vi "write.vi"(8 "error in (no error)":errorcluster, 10 "writeString":string, 11 "SerialReal in":refnum<class "SerialReal.lvclass">) -> (0 "error out":errorcluster, 3 "SerialReal out":refnum<class "SerialReal.lvclass">)   [LabVIEW 2013, in "SerialProtocols.lvlib" / "SerialReal.lvclass"]
uses:
  <userlib>/Common/SerialProtocols/SerialCommunicator/SerialReal/SerialReal.lvclass
  <userlib>/Common/SerialProtocols/SerialCommunicator/SerialReal/SerialReal.lvclass/SerialReal.ctl
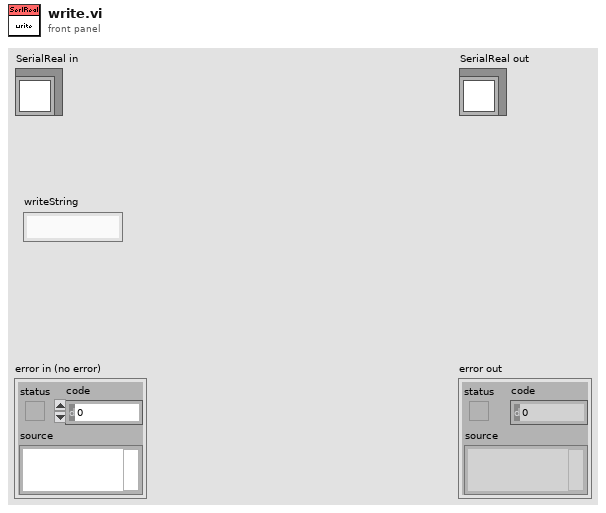
[diagram p1: front panel]
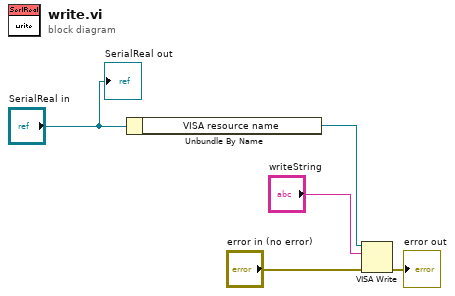
[diagram p0: block diagram]
diagram:
  n1 = Unbundle By Name("SerialReal in") -> ("VISA resource name"=w1:refnum<visa-resource-name>)
  n2 = VISA Write(VISA resource name=w1, write buffer="writeString", error in (no error)="error in (no error)") -> (error out=→"error out":errorcluster)  [unwired: 2 out]
  "SerialReal out" <- "SerialReal in"
